vi "Vision Processing.vi"(4 "error in (no error)":errorcluster) -> ()   [LabVIEW 2019]
doc: "This VI runs in parallel to other tasks. It gets images from the camera, processes them for color or shape and uses commands or globals to affect the behavior of other subsystems."
uses:
  Framework/Robot Global Data.vi
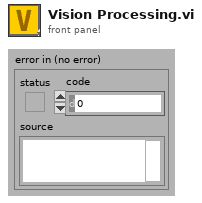
[diagram p1: front panel]
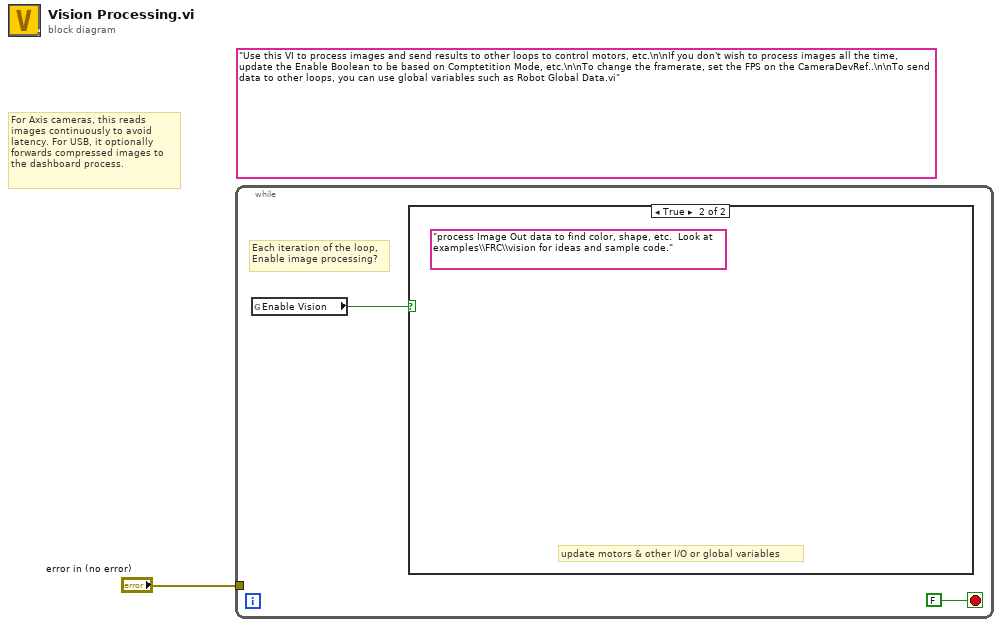
[diagram p0: block diagram]
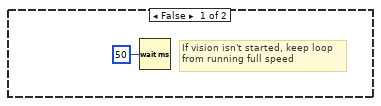
[diagram p2: hidden frame]
diagram:
  (unwired) "Use this VI to process images and send results to other loops to control motors, etc.\n\nIf you don't wish to process images all the time, update the Enable Boolean to be based on Comptetition Mode, etc.\n\nTo change the framerate, set the FPS on the CameraDevRef..\n\nTo send data to other loops, you can use global variables such as Robot Global Data.vi"
  # "For Axis cameras, this reads\nimages continuously to avoid\nlatency. For USB, it optionally\nforwards compressed images to\nthe dashboard process."
  n1 = while {
    tunnel: "error in (no error)" -> [_]
    stop <- FALSE stop-if-true
    # "Each iteration of the loop,\nEnable image processing?"
    n2 = global read "Robot Global Data.vi" "Enable Vision"() -> (w2:bool)
    n3 = case shown="True" w2 {
      frame False {
        # "If vision isn't started, keep loop\nfrom running full speed"
        n4 = Wait (ms)(milliseconds to wait=u32 50) -> ()  [unwired: 1 out]
      }
      frame True {
        (unwired) "process Image Out data to find color, shape, etc.  Look at examples\\FRC\\vision for ideas and sample code."
        # "update motors & other I/O or global variables"
      }
    }
  }
